vi "NI_Security Constants.vi"(11 "index in":T1(ring) caption="索引输入") -> (3 "msg out":string caption="消息输出")   [LabVIEW 2016]
panel:
  in  "constants":string[](array[string])=["%s \\n错误代码： %d \\n%s", "无法登录", "无法找到任何NI域", "无法更改密码"] caption="常量"
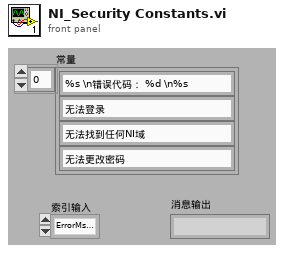
[diagram p1: front panel]
types:
  T1 = enum16{"ErrorMsgTemplate", "UnableToLogin", "UnableToFindDomain", "UnableToChangePasswd"}
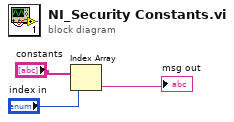
[diagram p0: block diagram]
diagram:
  n1 = Index Array(array="constants", index="index in") -> (element=→"msg out":string)
